vi "C1G2_Assemble Query.vi"(7 "Symbol Rate":dbl=500000.0 format="%#_6p", 8 "RFID":bool, 9 "Parameters Query":T2={"DR"=FALSE, "M"=1, "TRext (T=Pilot Tone)"=FALSE, "Sel"=1, "Session"=0, "Q"=0, "Target"=FALSE} {"Session" items=["S0", "S1", "S2", "S3"]; "Sel" items=["All", "All2", "~SL", "SL"]; "M" items=["M=1", "M=2", "M=4", "M=8"]}, 10 "Parameters Select":T3={"Target"=0, "Action"=0, "MemBank"=1, "truncate"=FALSE} {"MemBank" items=["00 RFU", "01 EPC", "10 TID", "11 User"]; "Action" items=["000", "001", "010", "011", "100", "101", "110", "111"]; "Target" items=["000 Inventoried (S0)", "001 Inventoried (S1)", "010 Inventoried (S2)", "011 Inventoried (S3)", "100 SL", "101 RFU", "110 RFU", "111 RFU"]}, 11 "Parameters Symbols":T1={"Tari"=8e-06, "PW"=0.5, "factor for \"1\" symbol"=0.5, "RTcal"=2.5, "TRcal"=3.0, "Delimiter"=1.25e-05} {"TRcal" min=1.1 max=3.0 step=0.1; "RTcal" min=2.5 max=3.0 step=0.1; "factor for \"1\" symbol" min=0.5 max=1.0 step=0.1; "PW" min=0.265 max=0.525 step=0.001; "Tari" format="%#_3p"}) -> (2 "Signal out":u8[](array[numeric]))   [LabVIEW 2015]
panel:
  in  "Select":bool
  out "CRC-16":u8[](array[numeric])=[1, 0, 1, 1, 0, 0, 0, 0, 0, 0, 0, 0, 0, 0, 0, 0] format="%0x"
  out "Query":i32
  out "CW":i32
  out "Sym0":i32
  out "Sym1":i32
  out "CRC-5":bool[](array[boolean])
  out "CRC-5":u8[](array[numeric])=[1, 0, 1, 1, 0] format="%0x"
  out "Symbols":i32=53374
  out "Digital Waveform":waveform(u8)(graph)={"t0"=timestamp(0 s since 1904-01-01), "dt"=1e-07, "Y"=array[53374 elements]}
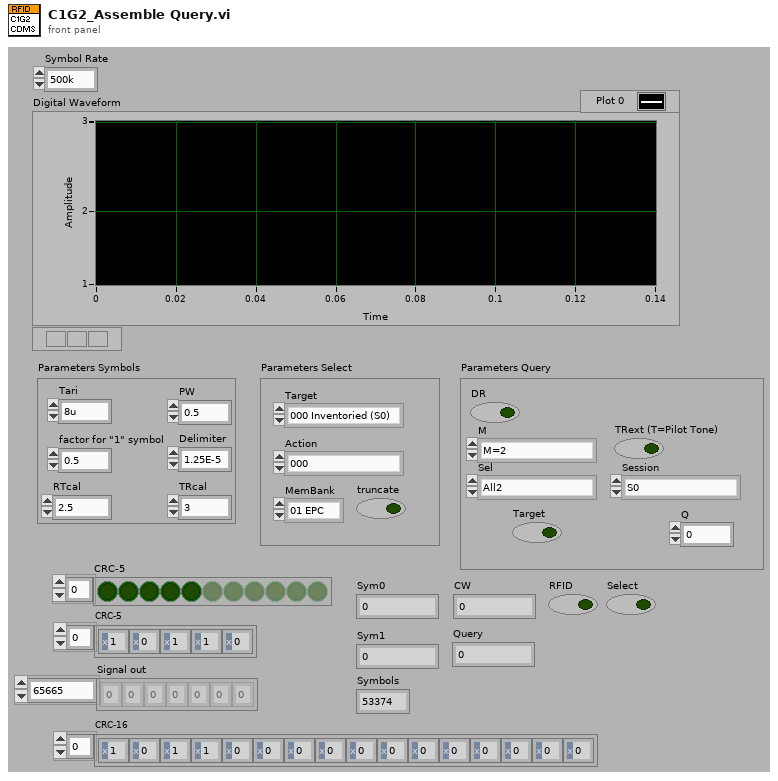
[diagram p1: front panel]
types:
  T1 = cluster{"Tari":dbl, "PW":dbl, "factor for \"1\" symbol":dbl, "RTcal":dbl, "TRcal":dbl, "Delimiter":dbl}
  T2 = cluster{"DR":bool, "M":u16, "TRext (T=Pilot Tone)":bool, "Sel":u16, "Session":u16, "Q":u8, "Target":bool}
  T3 = cluster{"Target":u16, "Action":u16, "MemBank":u16, "truncate":bool}
  T4 = typedef "C1G2_BasicsData.ctl" = cluster{"Symbol \"0\"":u8[], "Symbol \"1\"":u8[], "RT Preamble":u8[], "RT Frame Sync":u8[], "Sample Rate":dbl, "LOW-Pulse":u8[], "HIGH-Pulse":u8[], "RT cal":u8[]}
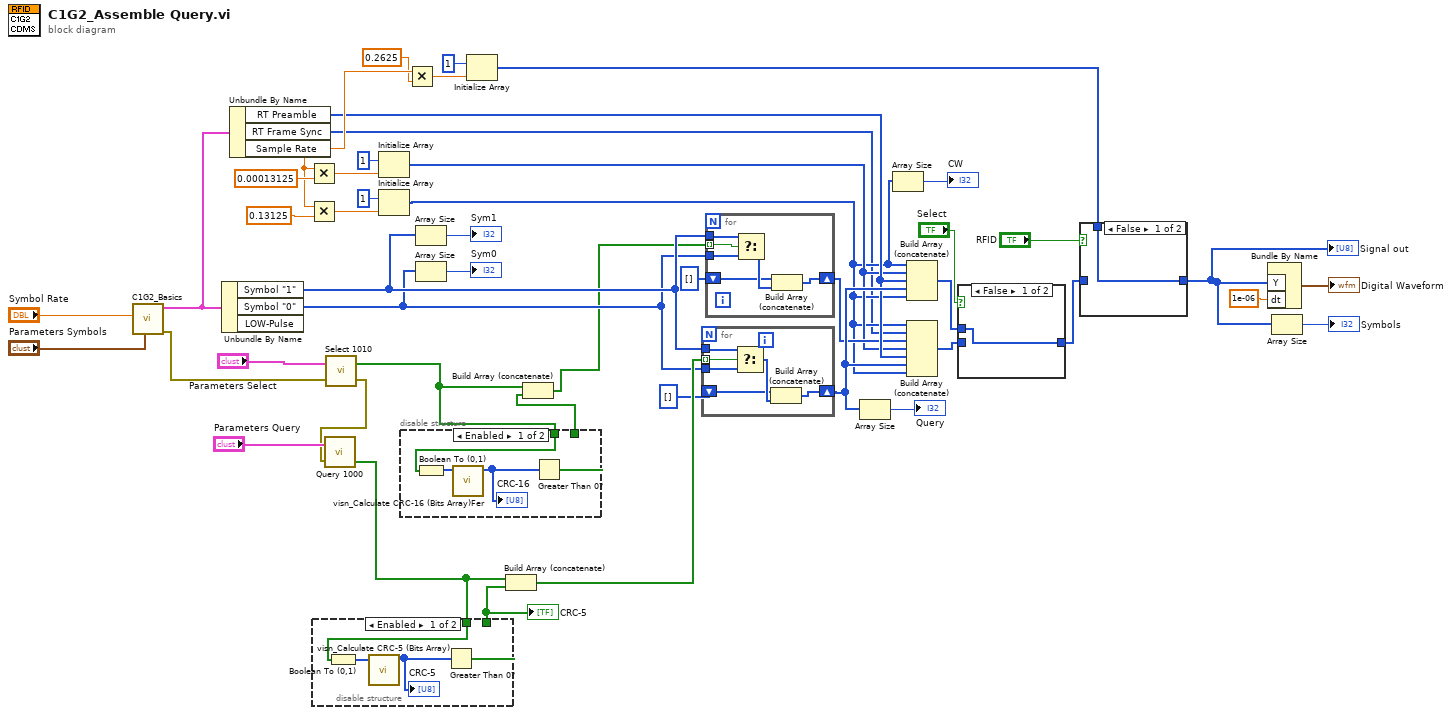
[diagram p0: block diagram]
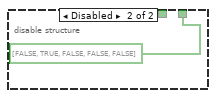
[diagram p4: hidden frame]
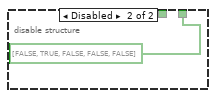
[diagram p5: hidden frame]
diagram:
  n1 = call "C1G2_Basics.vi"("Parameters Symbols"="Parameters Symbols", "Symbol Rate"="Symbol Rate") -> ("error out"=w31:errorcluster, "Basic Components"=w33:T4)  [unwired: 8 in]
  n2 = Unbundle By Name(w33) -> ("Symbol \"1\""=w27:u8[], "Symbol \"0\""=w25:u8[])  [unwired: 1 out]
  n3 = Unbundle By Name(w33) -> ("RT Preamble"=w9:u8[], "RT Frame Sync"=w1:u8[], "Sample Rate"=w17:dbl)
  n4 = Multiply(x=w17, y=0.00013125 ("Pause length /s")) -> (x*y=w40:dbl)
  n5 = Multiply(x=w17, y=0.13125 ("Pause length /s")) -> (x*y=w36:dbl)
  n6 = call "Select 1010.vi"("error in (no error)"=w31, "Parameters Select"="Parameters Select") -> ("error out"=w30:errorcluster, "Array"=w18:bool[])
  n7 = call "Query 1000.vi"("error in (no error)"=w30, "Parameters Query"="Parameters Query") -> ("Array"=w21:bool[])  [unwired: 1 out]
  n8 = disable-structure shown="Enabled" {
    disable-tunnel: w21 -> [w50 _]
    disable-tunnel: [w48 bool[] [FALSE, TRUE, FALSE, FALSE, FALSE]] -> w32
    frame Enabled {
      n9 = Boolean To (0,1)(Boolean=w50) -> (0, 1=w51:i16[])
      n10 = call "visn_Calculate CRC-5 (Bits Array).vi"("Bits Array"=w51) -> ("CRC-5"=w49:u8[])  [unwired: 10 in]
      "CRC-5" <- w49
      n11 = Greater Than 0?(x=w49) -> (x > 0?=w48:bool[])
    }
    frame Disabled {
    }
  }
  "CRC-5" <- w32
  n12 = Initialize Array(u8 1 ("element"), w40) -> (w7:u8[])
  n13 = Initialize Array(u8 1 ("element"), w36) -> (w2:u8[])
  n14 = disable-structure shown="Enabled" {
    disable-tunnel: w18 -> [w56 _]
    disable-tunnel: [w55 bool[] [FALSE, TRUE, FALSE, FALSE, FALSE]] -> w20
    frame Enabled {
      n15 = Boolean To (0,1)(Boolean=w56) -> (0, 1=w54:i16[])
      n16 = call "visn_Calculate CRC-16 (Bits Array)Fer.vi"("Bits Array"=w54) -> ("CRC-16"=w53:u8[])  [unwired: 10 in]
      "CRC-16" <- w53
      n17 = Greater Than 0?(x=w53) -> (x > 0?=w55:bool[])
    }
    frame Disabled {
    }
  }
  n18 = Multiply(x=w17, y=0.2625 ("Pause length /s")) -> (x*y=w15:dbl)
  n19 = Array Size(array=w27) -> (size(s)=→"Sym1":i32)
  n20 = Array Size(array=w25) -> (size(s)=→"Sym0":i32)
  n21 = Initialize Array(u8 1 ("element"), w15) -> (w11:u8[])
  n22 = Build Array (concatenate)(w21, w32) -> (w29:bool[])
  n23 = Build Array (concatenate)(w18, w20) -> (w19:bool[])
  n24 = for {
    tunnel: w29 -> [w63] mode=indexing
    tunnel: w25 -> [w61]
    tunnel: w27 -> [w62]
    shift-right: [w60] -> w10
    shift-left: u8[] [] ("s? t:f") -> [w58]
    n25 = Select(t=w62, s=w63, f=w61) -> (s? t:f=w59:u8[])
    n26 = Build Array (concatenate)(w58, w59) -> (w60:u8[])
  }
  n27 = for {
    tunnel: w19 -> [w69] mode=indexing
    tunnel: w25 -> [w67]
    tunnel: w27 -> [w68]
    shift-right: [w66] -> w8
    shift-left: u8[] [] ("s? t:f") -> [w64]
    n28 = Select(t=w68, s=w69, f=w67) -> (s? t:f=w65:u8[])
    n29 = Build Array (concatenate)(w64, w65) -> (w66:u8[])
  }
  n30 = Array Size(array=w10) -> (size(s)=→"Query":i32)
  n31 = Array Size(array=w2) -> (size(s)=→"CW":i32)
  n32 = Build Array (concatenate)(w2, w7, w9, w10, w2) -> (w6:u8[])
  n33 = Build Array (concatenate)(w2, w1, w8, w7, w9, w10, w2) -> (w5:u8[])
  n34 = case shown="False" "Select" {
    tunnel: w5 -> [_ w71]
    tunnel: [w70 w71] -> w3
    tunnel: w6 -> [w70 _]
    frame False {
    }
    frame True {
    }
  }
  n35 = case shown="False" "RFID" {
    tunnel: w3 -> [_ w73]
    tunnel: [w72 w73] -> w12
    tunnel: w11 -> [w72 _]
    frame False {
    }
    frame True {
    }
  }
  "Signal out" <- w12
  n36 = Bundle By Name("Y"=w12, "dt"=1e-06) -> (→"Digital Waveform":waveform(u8))  [unwired: 1 in]
  n37 = Array Size(array=w12) -> (size(s)=→"Symbols":i32)
